vi "dashboard.vi"() -> ()   [LabVIEW 2013]
panel:
  out "Drive":string="NORMAL"
  out "Catapult Puller":string="???"
  out "Intake":string="???"
  out "Electromagnet":bool
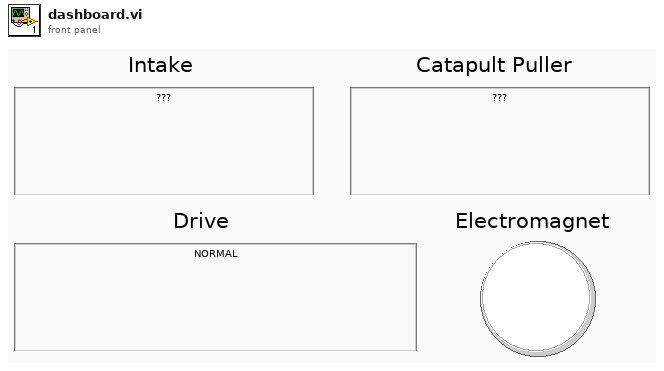
[diagram p1: front panel]
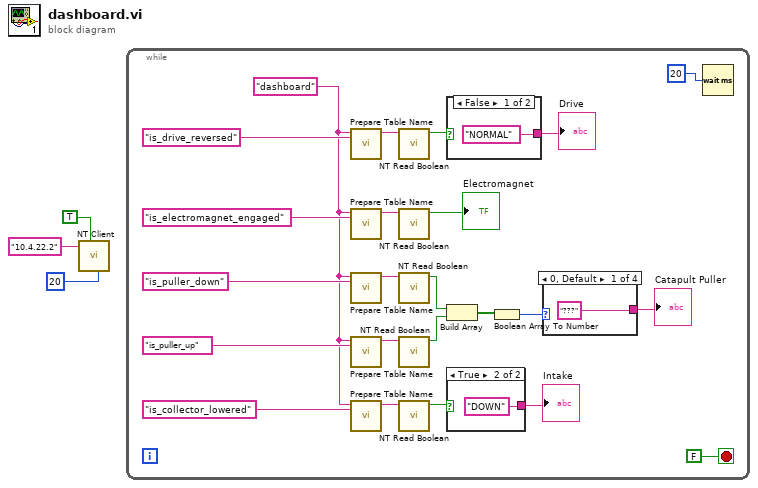
[diagram p0: block diagram]
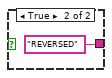
[diagram p2: hidden frame]
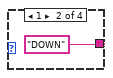
[diagram p3: hidden frame]
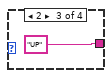
[diagram p4: hidden frame]
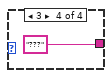
[diagram p5: hidden frame]
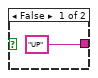
[diagram p6: hidden frame]
diagram:
  n1 = call <vilib>:"NT Client.vi"("Update Time"=20, "Automatic restart"=TRUE, "Server IP Address"="10.4.22.2") -> ()  [unwired: 9 in]
  n2 = while {
    stop <- FALSE stop-if-true
    w5 = "dashboard"
    n3 = call <vilib>:"Prepare Table Name.vi"("Name"="is_drive_reversed", "Table Prefix"=w5) -> ("Prefixed Name"=w7:string)  [unwired: 9 in]
    n4 = call <vilib>:"Prepare Table Name.vi"("Name"="is_electromagnet_engaged", "Table Prefix"=w5) -> ("Prefixed Name"=w24:string)  [unwired: 9 in]
    n5 = call <vilib>:"Prepare Table Name.vi"("Name"="is_puller_down", "Table Prefix"=w5) -> ("Prefixed Name"=w17:string)  [unwired: 9 in]
    n6 = call <vilib>:"Prepare Table Name.vi"("Name"="is_puller_up", "Table Prefix"=w5) -> ("Prefixed Name"=w15:string)  [unwired: 9 in]
    n7 = call <vilib>:"Prepare Table Name.vi"("Name"="is_collector_lowered", "Table Prefix"=w5) -> ("Prefixed Name"=w21:string)  [unwired: 9 in]
    n8 = call <vilib>:"NT Read Boolean.vi"("Name"=w7) -> ("Boolean"=w6:bool)  [unwired: 9 in, 1 out]
    n9 = call <vilib>:"NT Read Boolean.vi"("Name"=w24) -> ("Boolean"=→"Electromagnet":bool)  [unwired: 9 in, 1 out]
    n10 = call <vilib>:"NT Read Boolean.vi"("Name"=w17) -> ("Boolean"=w14:bool)  [unwired: 9 in, 1 out]
    n11 = call <vilib>:"NT Read Boolean.vi"("Name"=w15) -> ("Boolean"=w13:bool)  [unwired: 9 in, 1 out]
    n12 = call <vilib>:"NT Read Boolean.vi"("Name"=w21) -> ("Boolean"=w20:bool)  [unwired: 9 in, 1 out]
    n13 = case shown="False" w6 {
      tunnel: ["NORMAL" "REVERSED"] -> w4
      frame False {
      }
      frame True {
      }
    }
    "Drive" <- w4
    n14 = Build Array(w14, w13) -> (w12:bool[])
    n15 = case shown="True" w20 {
      tunnel: ["UP" "DOWN"] -> w19
      frame False {
      }
      frame True {
      }
    }
    "Intake" <- w19
    n16 = Boolean Array To Number(Boolean array=w12) -> (number=w11:u32)
    n17 = case shown="0, Default" w11 {
      tunnel: ["???" "DOWN" "UP" "???"] -> w10
      frame 0, Default {
      }
      frame 1 {
      }
      frame 2 {
      }
      frame 3 {
      }
    }
    "Catapult Puller" <- w10
    n18 = Wait (ms)(milliseconds to wait=u32 20) -> ()  [unwired: 1 out]
  }
